vi "Register Control.vi"(8 "error in (no error)":errorcluster, 9 "Control ref":refnum<vi>, 10 "Control":T1, 11 "ATM View Model in":refnum<class "ATM View Model.lvclass">) -> (0 "error out":errorcluster, 3 "ATM View Model out":refnum<class "ATM View Model.lvclass">)   [LabVIEW 2020, in "ATM View Model.lvclass"]
uses:
  ATM View Model.lvclass
  Controls.ctl
  ATM View Model.lvclass/ATM View Model.ctl
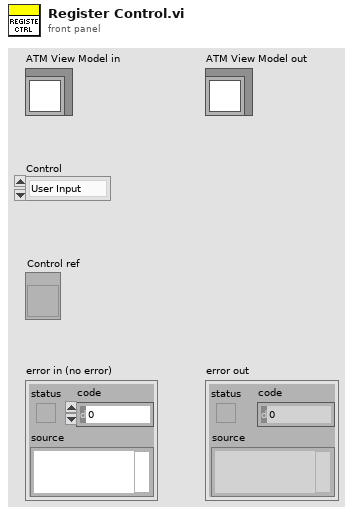
[diagram p1: front panel]
types:
  T1 = typedef "ATM View Model.lvclass/Controls.ctl" = enum16{"User Input", "Enter", "Left Menu", "Righ Menu", "Left Button", "Right Button", "Card Simulator"}
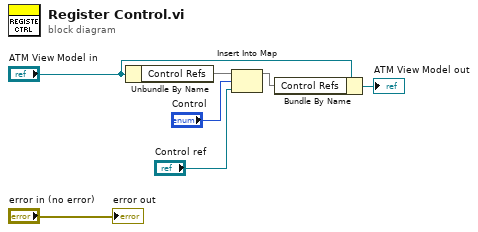
[diagram p0: block diagram]
diagram:
  n1 = Unbundle By Name("ATM View Model in") -> ("Control Refs"=w4:map{T1, refnum<vi>})
  n2 = Insert Into Map(map in=w4, key="Control", value="Control ref") -> (map out=w3:map{T1, refnum<vi>})  [unwired: 2 out]
  n3 = Bundle By Name(cluster="ATM View Model in", "Control Refs"=w3) -> (→"ATM View Model out":refnum<class "ATM View Model.lvclass">)
  "error out" <- "error in (no error)"
